vi "Host_rasterScanning.vi"() -> ()   [LabVIEW 2017]
uses:
  <vilib>/FPGAPlugInAG/cRIO-9082/niLvFpga_Open_cRIO-9082.vi
  <vilib>/rvi/interface/common/dynamic/niFpgaDynamicAddResources.vi
  <vilib>/FPGAPlugInAG/Dynamic/niLvFpga_Reset_Dynamic.vi
  <vilib>/Utility/error.llb/Error Cluster From Error Code.vi
  <vilib>/rvi/errors/niLvFpgaAdjustHostInterfaceError.vi
  <vilib>/rvi/interface/common/niFpgaWaitOnOcc.vi
  <vilib>/FPGAPlugInAG/Dynamic/niLvFpga_Run_Dynamic.vi
  <vilib>/Utility/file.llb/Write To Spreadsheet File (DBL).vi
  <vilib>/rvi/interface/nirviOpenFPGA/nirviOpenFPGA.xnode
  FPGA Bitfiles/simpletest_FPGATarget_rasterScanning_--ABLWds12k.lvbitx
  <vilib>/rvi/interface/nirviMethod/nirviMethod.xnode
  <vilib>/rvi/interface/nirviReadWriteControl/nirviReadWriteControl.xnode
  <vilib>/rvi/interface/Simulation/niFpgaSimulationCallBeginRW.vi
  <vilib>/rvi/errors/niLvFpgaMergeErrorWithErrorCode.vi
  <vilib>/FPGAPlugInAG/Dynamic/niLvFpga_ConfigureFifo_Dynamic.vi
  <vilib>/FPGAPlugInAG/Dynamic/niLvFpga_StartFifo_Dynamic.vi
  NiFpgaLv.dll
  <vilib>/FPGAPlugInAG/Dynamic/niLvFpga_ReadFifo_Dynamic.vi
panel:
  out "z output":dbl=3.606201171875
  out "y output":dbl=6.347320556640625
  out "x output":dbl=-2.883392333984375
  out "deflection":dbl=0.0245361328125
  out "z":dbl=-5.92041015625
  out "y":dbl=4.91998291015625
  out "x":dbl=0.027740478515625
  out "Elements Remaining":u32
  out "FINISH_SIGNAL":bool
  in  "stop":bool
  in  "Threshold":T1={"x threshold"=0.02301025390625, "y threshold"=0.02301025390625, "z threshold"=0.5, "deflection threshold"=0.024993896484375}
  in  "ImageToSample":T2={"image size_x"=512, "image size_y"=512, "sample start_x"=0.0, "sample start_y"=0.0, "sample end_x"=6.0, "sample end_y"=6.0}
  in  "deflection control":T3={"SetPoint (V)"=0.0, "scanning I"=500.0, "scanning P"=0.0146484375, "Initial I (V)"=0.0, "Upper Limit (V)"=9.900000095367432, "Lower Limit (V)"=-9.900000095367432}
  in  "z control":T4={"SetPoint (V)"=-2.0, "I"=100.0, "P"=0.0595703125, "Initial I (V)"=0.0, "Upper Limit (V)"=9.900000095367432, "Lower Limit (V)"=-9.900000095367432}
  in  "y control":T3={"SetPoint (V)"=0.0, "scanning I"=1850.0, "scanning P"=0.08984375, "Initial I (V)"=0.0, "Upper Limit (V)"=9.900000095367432, "Lower Limit (V)"=-9.900000095367432}
  in  "x control":T3={"SetPoint (V)"=0.0, "scanning I"=1850.0, "scanning P"=0.08984375, "Initial I (V)"=0.0, "Upper Limit (V)"=9.900000095367432, "Lower Limit (V)"=-9.900000095367432}
  in  "Clock (uSec)":T5={"XY Clock (uSec)"=20.0, "Z Clock (uSec)"=3.0, "Stage Clock (uSec)"=500.0, "Scan Clock (uSec)"=10.0, "Sampling Clock (uSec)"=6500.0, "pixel segment"=512000}
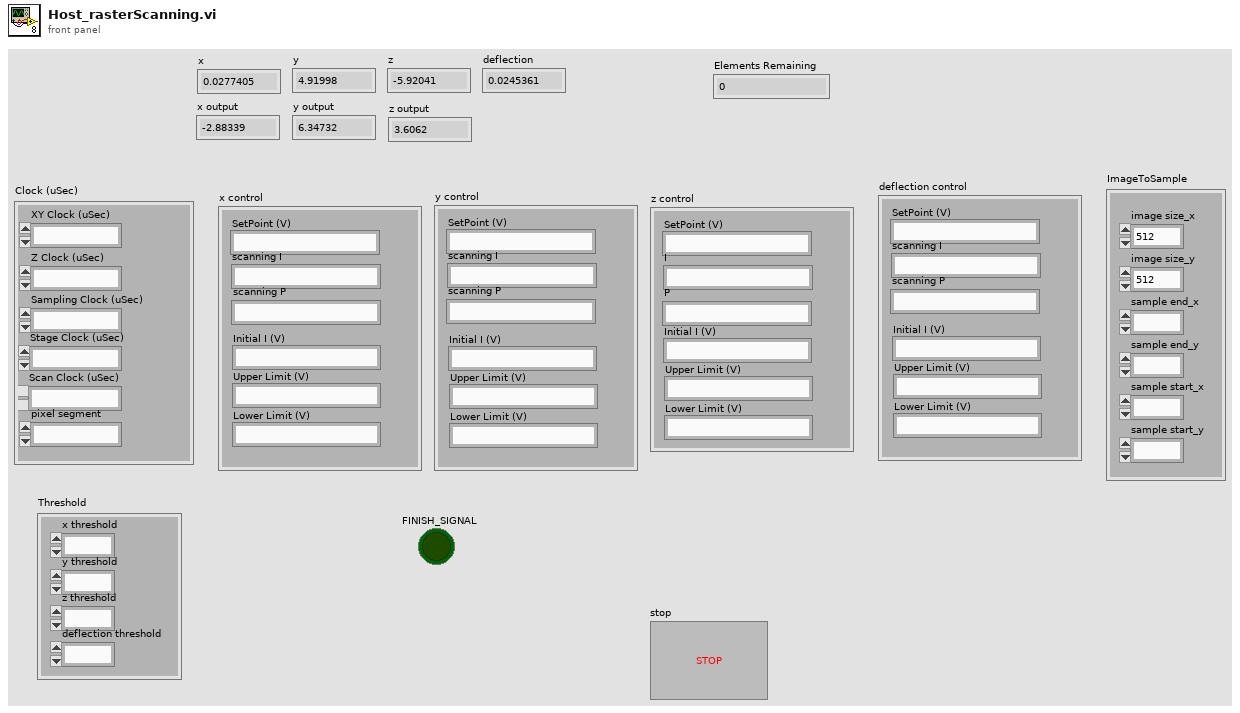
[diagram p1: front panel]
types:
  T1 = cluster{"x threshold":fxp<+/-,20,5>, "y threshold":fxp<+/-,20,5>, "z threshold":fxp<+/-,20,5>, "deflection threshold":fxp<+/-,20,5>}
  T2 = cluster{"image size_x":u16, "image size_y":u16, "sample start_x":fxp<+/-,26,5>, "sample start_y":fxp<+/-,26,5>, "sample end_x":fxp<+/-,26,5>, "sample end_y":fxp<+/-,26,5>}
  T3 = cluster{"SetPoint (V)":fxp<+/-,26,5>, "scanning I":fxp<+,21,13>, "scanning P":fxp<+,15,5>, "Initial I (V)":fxp<+/-,10,5>, "Upper Limit (V)":fxp<+/-,26,5>, "Lower Limit (V)":fxp<+/-,26,5>}
  T4 = cluster{"SetPoint (V)":fxp<+/-,26,5>, "I":fxp<+,21,13>, "P":fxp<+,15,5>, "Initial I (V)":fxp<+/-,10,5>, "Upper Limit (V)":fxp<+/-,26,5>, "Lower Limit (V)":fxp<+/-,26,5>}
  T5 = cluster{"XY Clock (uSec)":fxp<+,32,32>, "Z Clock (uSec)":fxp<+,32,32>, "Stage Clock (uSec)":fxp<+,32,32>, "Scan Clock (uSec)":fxp<+,32,32>, "Sampling Clock (uSec)":fxp<+,32,32>, "pixel segment":u32}
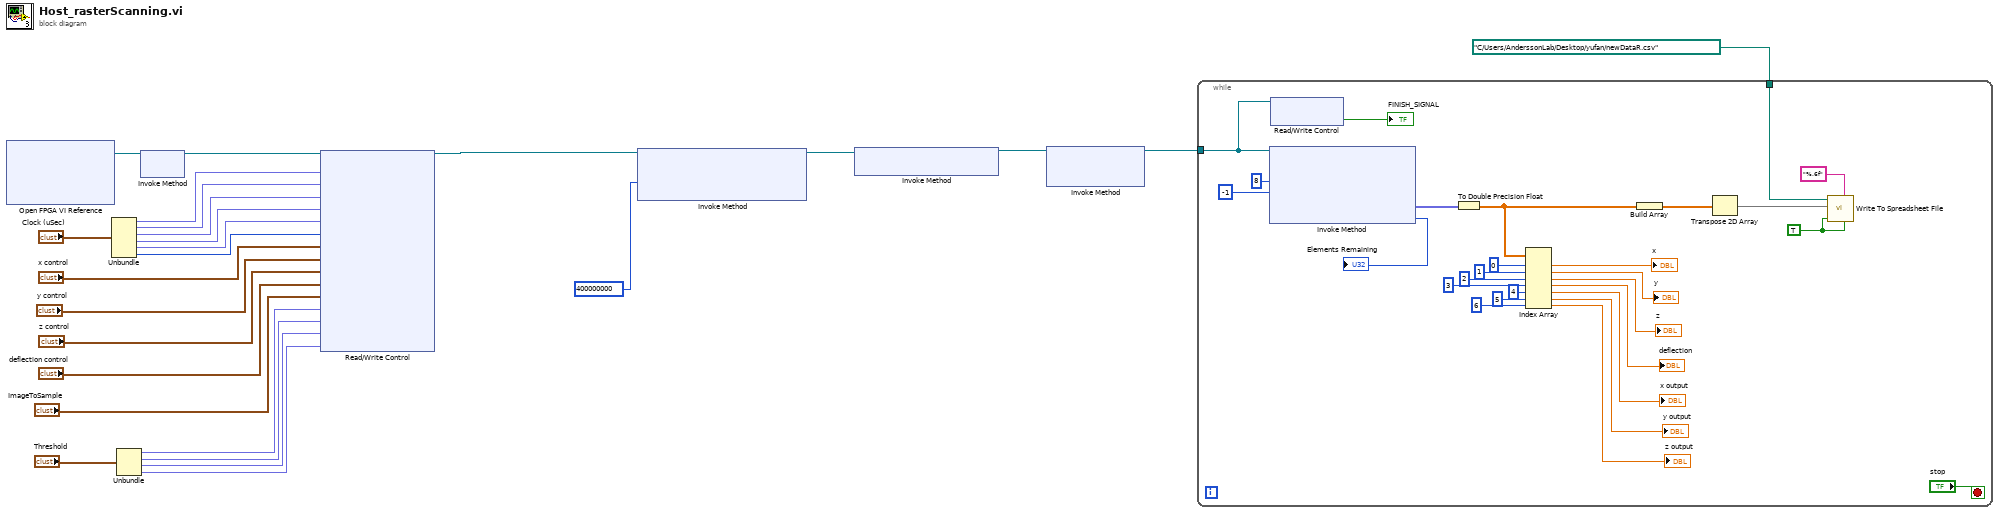
[diagram p0: block diagram]
diagram:
  n1 = xnode "Open FPGA VI Reference"() -> ("FPGA VI Reference Out"=w25:refnum<k20>)  [unwired: 2 in, 1 out]
  n2 = Unbundle("Clock (uSec)") -> ("XY Clock (uSec)"=w22:fxp<+,32,32>, "Z Clock (uSec)"=w21:fxp<+,32,32>, "Stage Clock (uSec)"=w20:fxp<+,32,32>, "Scan Clock (uSec)"=w19:fxp<+,32,32>, "Sampling Clock (uSec)"=w18:fxp<+,32,32>, "pixel segment"=w17:u32)
  n3 = Unbundle("Threshold") -> ("x threshold"=w10:fxp<+/-,20,5>, "y threshold"=w9:fxp<+/-,20,5>, "z threshold"=w8:fxp<+/-,20,5>, "deflection threshold"=w7:fxp<+/-,20,5>)
  n4 = xnode "Invoke Method"("FPGA VI Reference In"=w25) -> ("FPGA VI Reference Out"=w24:refnum<k20>)  [unwired: 1 in, 1 out]
  n5 = xnode "Read/Write Control"("FPGA VI Reference In"=w24, "XY Clock (uSec)"=w22, "Z Clock (uSec)"=w21, "Stage Clock (uSec)"=w20, "Scan Clock (uSec)"=w19, "Sampling Clock (uSec)"=w18, "pixel segment"=w17, "x control"="x control", "y control"="y control", "z control"="z control", "deflection control"="deflection control", "ImageToSample"="ImageToSample", "x threshold"=w10, "y threshold"=w9, "z threshold"=w8, "deflection threshold"=w7) -> ("FPGA VI Reference Out"=w1:refnum<k20>)  [unwired: 1 in, 1 out]
  n6 = xnode "Invoke Method"("FPGA VI Reference In"=w1, "Requested Depth"=u32 400000000) -> ("FPGA VI Reference Out"=w5:refnum<k20>)  [unwired: 1 in, 2 out]
  n7 = xnode "Invoke Method"("FPGA VI Reference In"=w5) -> ("FPGA VI Reference Out"=w4:refnum<k20>)  [unwired: 1 in, 1 out]
  n8 = xnode "Invoke Method"("FPGA VI Reference In"=w4) -> ("FPGA VI Reference Out"=w3:refnum<k20>)  [unwired: 2 in, 1 out]
  n9 = while {
    tunnel: w3 -> [w51]
    tunnel: path "C:/Users/AnderssonLab/Desktop/yufan/newDataR.csv" ("file path (dialog if empty)") -> [w26]
    stop <- "stop" stop-if-true
    w31 = TRUE
    n10 = xnode "Invoke Method"("FPGA VI Reference In"=w51, "Number of Elements"=u32 8, "Timeout (ms)"=-1) -> ("Data"=w39:fxp<+/-,25,5>[], "Elements Remaining"=→"Elements Remaining":u32)  [unwired: 1 in, 2 out]
    n11 = xnode "Read/Write Control"("FPGA VI Reference In"=w51) -> ("signalToStop"=→"FINISH_SIGNAL":bool)  [unwired: 1 in, 2 out]
    n12 = To Double Precision Float(number=w39) -> (double precision float=w27:dbl[])
    n13 = Index Array(array=w27, index #1=0 ("index"), index #2=1 ("index"), index #3=2 ("index"), index #4=3 ("index"), index #5=4 ("index"), index #6=5 ("index"), index #7=6 ("index")) -> (element #1=→"x":dbl, element #2=→"y":dbl, element #3=→"z":dbl, element #4=→"deflection":dbl, element #5=→"x output":dbl, element #6=→"y output":dbl, element #7=→"z output":dbl)
    n14 = Build Array(w27) -> (w29:dbl[][])
    n15 = Transpose 2D Array(2D array=w29) -> (transposed array=w28:dbl[][])
    n16 = call-poly <vilib>:"Write To Spreadsheet File.vi"("transpose? (no:F)"=w31, "format (%.3f)"="%.6f", "append to file? (new file:F)"=w31, "2D data"=w28, "file path (dialog if empty)"=w26) -> ()  [unwired: 3 in, 1 out]
  }
